vi "Configure Offset Compensation.vi"(8 "error in (no error)":errorcluster, 9 "Function (0 : Voltage)":u16(ring) items=["Voltage", "Current", "Resistance"], 10 "Enable Compensation (T: Enable)":bool=TRUE, 11 "VISA resource name":refnum<visa-resource-name>) -> (0 "error out":errorcluster, 3 "VISA resource name out":refnum<visa-resource-name>)   [LabVIEW 2020, in "Keithley 2450.lvlib"]
doc: "Enables or disables offset compensation for measurements."
uses:
  Keithley 2450.lvlib
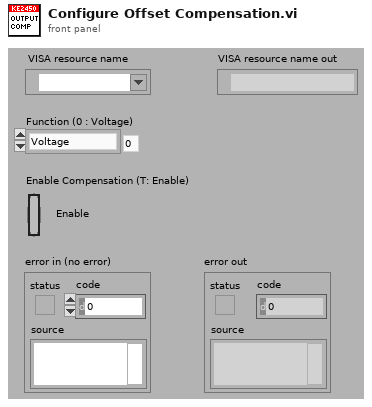
[diagram p1: front panel]
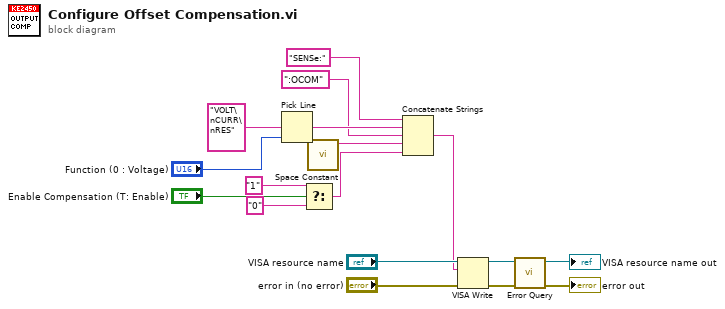
[diagram p0: block diagram]
diagram:
  n1 = Pick Line(multi-line string="VOLT\nCURR\nRES", line index="Function (0 : Voltage)") -> (output string=w10:string)  [unwired: 1 in]
  n2 = Select(t="1", s="Enable Compensation (T: Enable)", f="0") -> (s? t:f=w6:string)
  n3 = call <vilib>:"Space Constant.vi"() -> ("String"=w5:string)
  n4 = Concatenate Strings("SENSe:" ("string"), w10, ":OCOM" ("string"), w5, w6) -> (w8:string)
  n5 = VISA Write(VISA resource name="VISA resource name", write buffer=w8, error in (no error)="error in (no error)") -> (VISA resource name out=w4:refnum<visa-resource-name>, error out=w3:errorcluster)  [unwired: 1 out]
  n6 = call "Error Query.vi"("error in (no error)"=w3, "VISA resource name"=w4) -> ("error out"=→"error out":errorcluster, "VISA resource name out"=→"VISA resource name out":refnum<visa-resource-name>)  [unwired: 8 out]
